vi "Unit Test slice objects per SetSerializeSliceClass False.vi"() -> ()   [LabVIEW 2019, in "Sports Unit Tests.lvclass"]
uses:
  Sports Unit Tests.lvclass
  Classes/Sports Player/Sports Player.lvclass
  Classes/Tiger Woods/Tiger Woods.lvclass
  C:/DSCE code/Serialization/blueserializationdemo/Test/Sports/Classes/Human/Human.lvclass
  C:/DSCE code/Serialization/blueserializationdemo/Test/Sports/Classes/Sports Player/Sports Player.lvclass
  C:/DSCE code/Serialization/blueserializationdemo/Test/Sports/Classes/Golf Player/Golf Player.lvclass
  <userlib>/Blue Origin/BlueSerialization/BlueSerializer/SerializeOptions.ctl
  Classes/Human/Human.lvclass/Human.ctl
  Classes/Sports Player/Sports Player.lvclass/Sports Player.ctl
  Classes/Golf Player/Golf Player.lvclass/Golf Player.ctl
  Classes/Tiger Woods/Tiger Woods.lvclass/Tiger Woods.ctl
  Classes/Human/Write Age (years).vi
  Classes/Human/Write alive_.vi
  Classes/Human/Write Height (ft).vi
  Classes/Human/Write Name.vi
  Classes/Sports Player/Write Earnings (dollars).vi
  Classes/Sports Player/Write Professional_.vi
  Classes/Sports Player/Write Sponsor.vi
  Classes/Golf Player/Write # holes in one.vi
  Classes/Golf Player/Write League.vi
  Classes/Golf Player/Write longest drive (ft).vi
  Classes/Tiger Woods/Write # tantrums thrown.vi
  Classes/Tiger Woods/Write Current tour.vi
  Classes/Tiger Woods/Write Slice-To-This Class Name.vi
  <vilib>/Utility/error.llb/Clear Errors.vi
  <vilib>/addons/_JKI Toolkits/Caraya/classes/Test/Define Test.vi
  <vilib>/addons/_JKI Toolkits/Caraya/classes/Assert/Assert Equal Value_Variant.vi
  <vilib>/addons/_JKI Toolkits/Caraya/classes/Assert/Assert Not Error.vi
  <vilib>/addons/_JKI Toolkits/Caraya/classes/Assert/Assert.lvclass
  <userlib>/Blue Origin/BlueSerialization/BlueSerializer/BlueSerializer.lvclass
panel:
  out "Table":string[][](table)
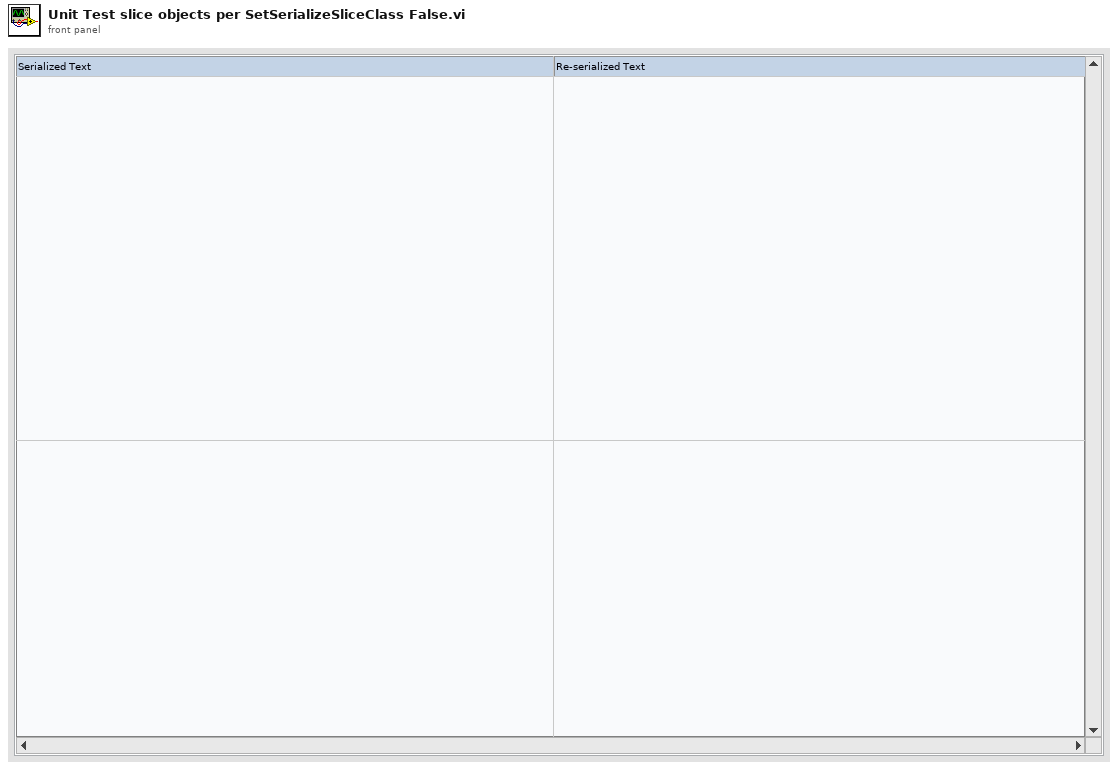
[diagram p1: front panel]
types:
  T1 = typedef "BlueSerialization.lvlib/BlueSerializer.lvclass/SerializeOptions.ctl" = cluster{"serialize non-BlueSerializable objects as hex?":bool, "slice objects per SetSerializeSliceClass.vi?":bool}
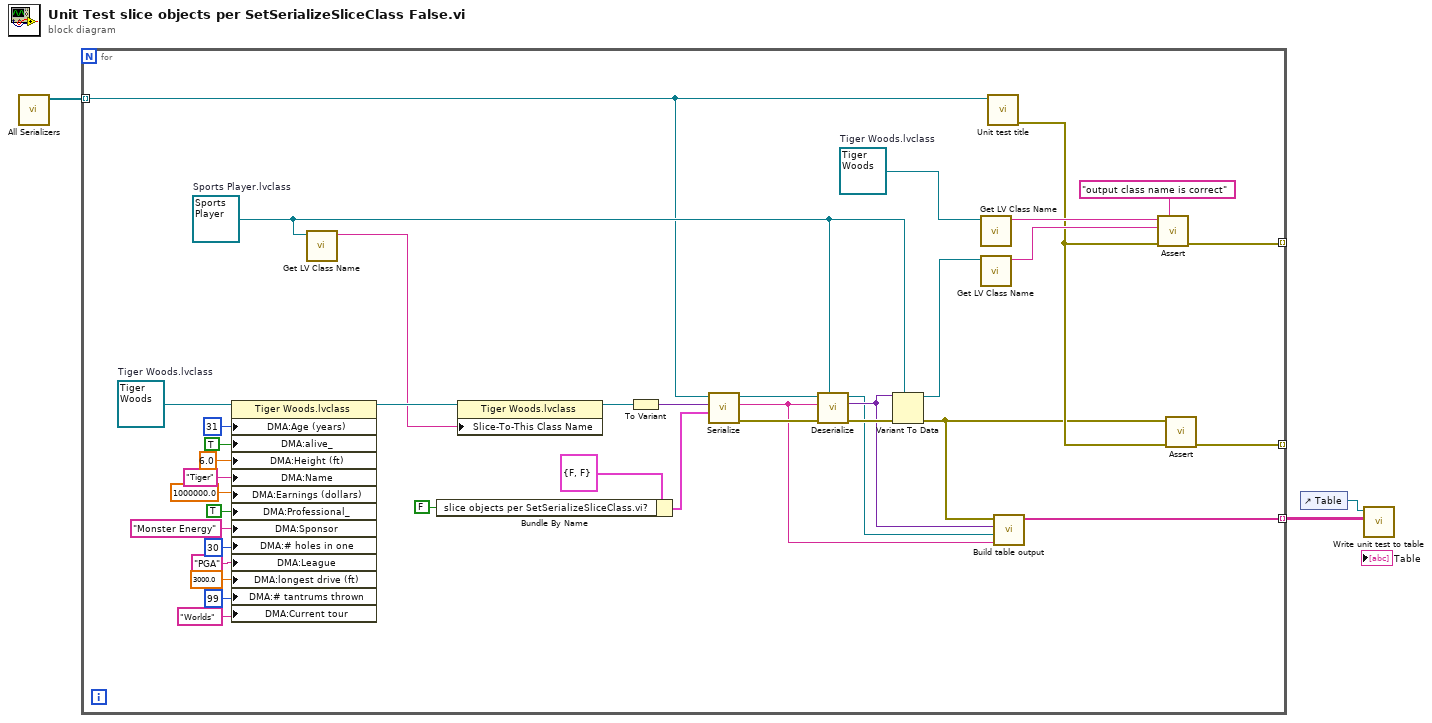
[diagram p0: block diagram]
diagram:
  n1 = call "All Serializers.vi"() -> ("All serializers"=w1:refnum<class "BlueSerializer.lvclass">[])  [unwired: 11 in]
  n2 = for {
    tunnel: w1 -> [w4] mode=indexing
    tunnel: [w8] -> w3 mode=indexing
    tunnel: [w13] -> _ mode=indexing
    tunnel: [w33] -> _ mode=indexing
    w15 = refnum<class "Tiger Woods.lvclass"> refnum  # Tiger Woods.lvclass
    w18 = refnum<class "Sports Player.lvclass"> refnum  # Sports Player.lvclass
    w32 = refnum<class "Tiger Woods.lvclass"> refnum  # Tiger Woods.lvclass
    n3 = property on="Property Node" class="Tiger Woods.lvclass"(reference=w32, "DMA:Age (years)"=u16 31 ("Age (years)"), "DMA:alive_"=TRUE ("alive_"), "DMA:Height (ft)"=6.0 ("Height (ft)"), "DMA:Name"="Tiger" ("Name"), "DMA:Earnings (dollars)"=1000000.0 ("Earnings (dollars)"), "DMA:Professional_"=TRUE ("Professional_"), "DMA:Sponsor"="Monster Energy" ("Sponsor"), "DMA:# holes in one"=30 ("# holes in one"), "DMA:League"="PGA" ("League"), "DMA:longest drive (ft)"=3000.0 ("longest drive (ft)"), "DMA:# tantrums thrown"=99 ("# tantrums thrown"), "DMA:Current tour"="Worlds" ("Current tour")) -> (reference out=w19:refnum<class "Tiger Woods.lvclass">)  [unwired: 1 in, 1 out]
    n4 = call <vilib>:"Get LV Class Name.vi"("object"=w18) -> ("class name"=w17:string)  [unwired: 9 in, 1 out]
    n5 = Bundle By Name(cluster=T1 {"serialize non-BlueSerializable objects as hex?"=FALSE, "slice objects per SetSerializeSliceClass.vi?"=FALSE} ("Serialize Options"), "slice objects per SetSerializeSliceClass.vi?"=FALSE ("Allow class slicing?")) -> (w5:T1)
    n6 = property class="Tiger Woods.lvclass"(reference=w19, "Slice-To-This Class Name"=w17) -> (reference out=w16:refnum<class "Tiger Woods.lvclass">)  [unwired: 1 in, 1 out]
    n7 = To Variant(anything=w16) -> (Variant=w39:variant)
    n8 = call <userlib>:"Serialize.vi"("Serialize Options"=w5, "Anything"=w39, "BlueSerializer in"=w4) -> ("error out"=w41:errorcluster, "Serialized Text"=w9:string, "BlueSerializer out"=w40:refnum<class "BlueSerializer.lvclass">)  [unwired: 6 in]
    n9 = call <userlib>:"Deserialize.vi"("Anything"=w18, "error in (no error)"=w41, "Serialized Text"=w9, "BlueSerializer in"=w40) -> ("error out"=w38:errorcluster, "Variant"=w11:variant, "BlueSerializer out"=w10:refnum<class "BlueSerializer.lvclass">)  [unwired: 5 in]
    n10 = Variant To Data(error in=w38, type=w18, Variant=w11) -> (data=w37:refnum<class "Sports Player.lvclass">, error out=w12:errorcluster)
    n11 = call <vilib>:"Get LV Class Name.vi"("object"=w15) -> ("class name"=w36:string)  [unwired: 9 in, 1 out]
    n12 = call <vilib>:"Get LV Class Name.vi"("object"=w37) -> ("class name"=w35:string)  [unwired: 9 in, 1 out]
    n13 = call "Unit test title.vi"("serializer"=w4) -> ("error out"=w14:errorcluster)  [unwired: 9 in, 1 out]
    n14 = call "Build table output.vi"("serialized text"=w9, "BlueSerializer in"=w10, "deserialized variant"=w11, "variant to data error"=w12) -> ("table output"=w8:string[])  [unwired: 7 in]
    n15 = call-poly <vilib>:"Assert.vi"("Label"="output class name is correct", "error in (no error)"=w14, "Y"=w35, "X"=w36) -> ("error out"=w33:errorcluster)  [unwired: 7 in]
    n16 = call-poly <vilib>:"Assert.vi"("error in (no error)"=w14, "Not Error?"=w12) -> ("error out"=w13:errorcluster)  [unwired: 9 in]
  }
  n17 = control-ref of="Table"() -> (w2:refnum<vi>)
  n18 = call "Write unit test to table.vi"("Table"=w3, "Table ref in"=w2) -> ()  [unwired: 9 in, 1 out]
